vi "Just practice array functions 2.vi"() -> ()   [LabVIEW 2020]
panel:
  out "appended array 2":dbl[](array[numeric])
  out "output array 2":dbl[](array[numeric])
  in  "Array 4":dbl[](array[numeric])
  out "appended array":dbl[][](array[numeric])
  in  "Array 3":dbl[](array[numeric])
  in  "Array 2":dbl[](array[numeric])
  out "output array":dbl[](array[numeric])
  in  "Array":dbl[][](array[numeric])
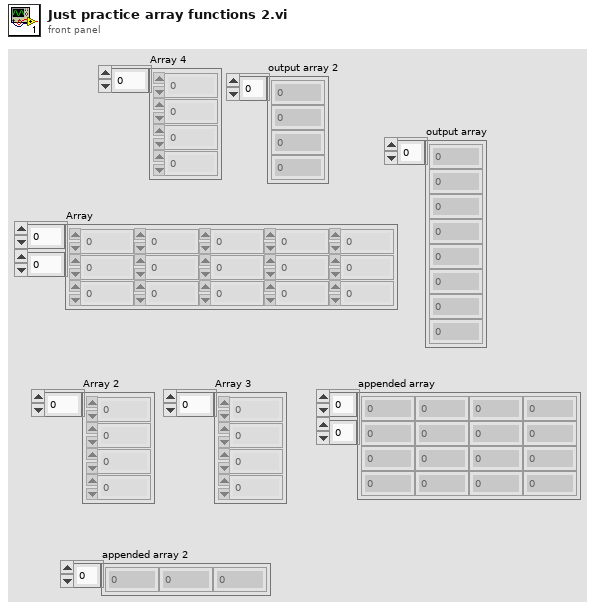
[diagram p1: front panel]
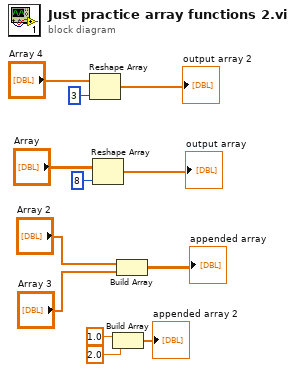
[diagram p0: block diagram]
diagram:
  n1 = Reshape Array "Reshape Array"("Array 4", 3 ("dimension size")) -> (→"output array 2":dbl[])
  n2 = Reshape Array "Reshape Array"("Array", 8 ("dimension size")) -> (→"output array":dbl[])
  n3 = Build Array(1.0 ("element"), 2.0 ("element")) -> (→"appended array 2":dbl[])
  n4 = Build Array "Build Array"("Array 2", "Array 3") -> (→"appended array":dbl[][])
